vi "array_repeats.vi"(10 "values_IN":dbl[](array[numeric])=[1.0, 2.0, 3.0, 4.0, 5.0, 6.0, 7.0, 8.0, 9.0, 10.0] format="%#_6p", 11 "repeats":i32=1 min=0) -> (2 "values_OUT":dbl[](array[numeric])=[1.0, 2.0, 3.0, 4.0, 5.0, 6.0, 7.0, 8.0, 9.0, 10.0] format="%#_6p")   [LabVIEW 2017, in "tools.lvlib"]
uses:
  tools.lvlib
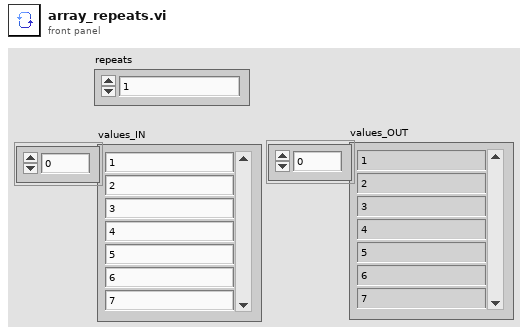
[diagram p1: front panel]
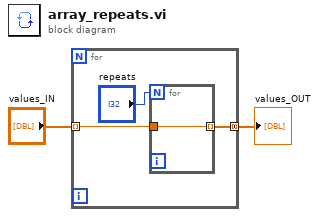
[diagram p0: block diagram]
diagram:
  n1 = for {
    tunnel: "values_IN" -> [w5] mode=indexing
    tunnel: [w3] -> w1 mode=concatenating
    n2 = for {
      N: "repeats" -> [_]
      tunnel: w5 -> [w6]
      tunnel: [w6] -> w3 mode=indexing
    }
  }
  "values_OUT" <- w1
